vi "Read Spec Page Path.vi"(8 "error in (no error)":errorcluster, 11 "IO PE Creation MDO in":refnum<class "ADAS_IO_Template_MDO.lvclass">) -> (0 "error out":errorcluster, 2 "Path to Spec Page VI":path, 3 "IO PE Creation MDO out":refnum<class "ADAS_IO_Template_MDO.lvclass">)   [LabVIEW 2020, in "ADAS_IO_Template_MDO.lvclass"]
uses:
  ADAS_IO_Template_MDO.lvclass
  ADAS_IO_Template_MDO.lvclass/ADAS_IO_Template_MDO.ctl
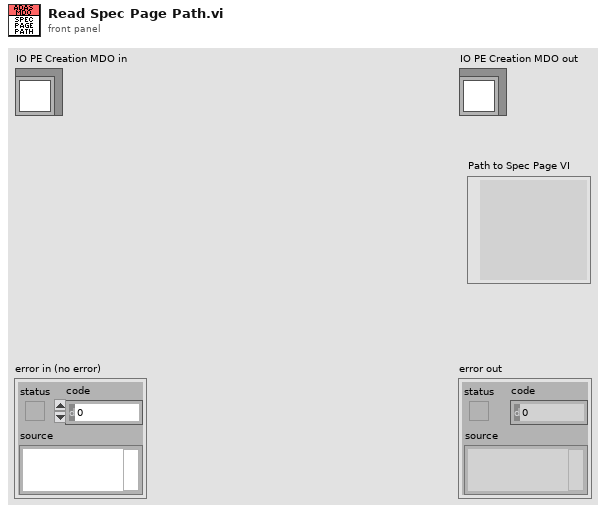
[diagram p1: front panel]
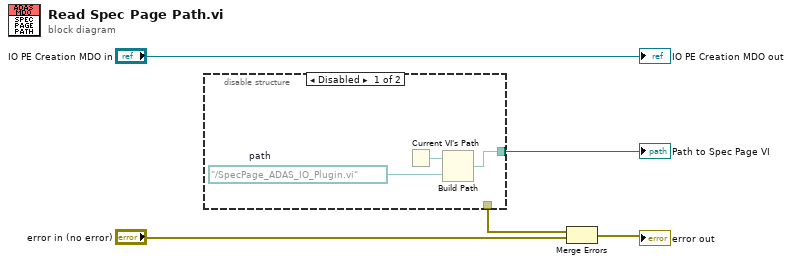
[diagram p0: block diagram]
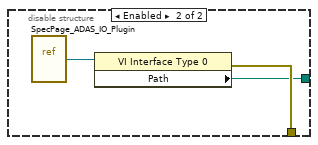
[diagram p2: hidden frame]
diagram:
  n1 = disable-structure shown="Disabled" {
    disable-tunnel: [w6 w9] -> w2
    disable-tunnel: [_ w10] -> w1
    frame Disabled {
      w7 = path "../SpecPage_ADAS_IO_Plugin.vi"  # path
      n2 = Current VI's Path() -> (path=w8:path)
      n3 = Build Path(base path=w8, name or relative path=w7) -> (appended path=w6:path)
    }
    frame Enabled {
      n4 = vi-ref "SpecPage_ADAS_IO_Plugin.vi"() -> (w11:refnum<vi>)
      n5 = property class="VI Interface Type 0"(reference=w11) -> (error out=w10:errorcluster, "Path"=w9:path)  [unwired: 1 in, 1 out]
    }
  }
  "Path to Spec Page VI" <- w2
  n6 = Merge Errors(w1, "error in (no error)") -> (→"error out":errorcluster)
  "IO PE Creation MDO out" <- "IO PE Creation MDO in"
